vi "InsertItemByPath.vi"(8 "error in (no error)":errorcluster, 9 "ILabVIEWItem in":refnum<class "ILabVIEWItem.lvclass">, 10 "Path":string, 11 "CDependencyList in":refnum<class "CDependencyList.lvclass">) -> (0 "error out":errorcluster, 3 "CDependencyList out":refnum<class "CDependencyList.lvclass">)   [LabVIEW 2020, in "DependencyInspection.lvlib" / "CDependencyList.lvclass"]
uses:
  CDependencyList.lvclass
  obj/Addons/LabVIEWObjectInterfaces.lvlibp/LabVIEWObjectInterfaces/ILabVIEWItem/ILabVIEWItem.lvclass
  CDependencyList.lvclass/CDependencyList.ctl
  <vilib>/Utility/miscctls.llb/LVMapReplaceAction.ctl
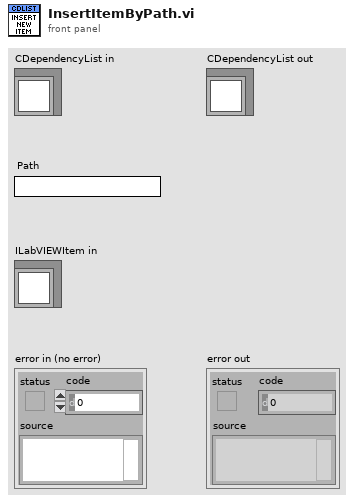
[diagram p1: front panel]
types:
  T1 = typedef "LVMapReplaceAction.ctl" = enum32{"Modify Entry only if found", "Add or Modify Entry", "Delete Entry"}
  T2 = typedef "DependencyInspection.lvlib/CDependencyList.lvclass/DependencyListRef.ctl" = refnum<data-value>
  T3 = typedef "DependencyInspection.lvlib/CDependencyList.lvclass/DependencyList.ctl" = map{string, refnum<class "ILabVIEWItem.lvclass">}
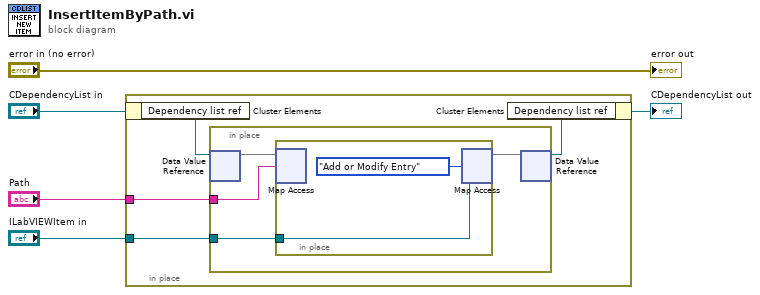
[diagram p0: block diagram]
diagram:
  n1 = in-place {
    in-place-border: "ILabVIEWItem in" -> [w9]
    in-place-border: "Path" -> [w6]
    n2 = in-place-cluster #1("CDependencyList in") -> ("Dependency list ref"=w8:T2)
    n3 = in-place {
      in-place-border: w9 -> [w13]
      in-place-border: w6 -> [w10]
      n4 = in-place-dvr #2(w8) -> (w12:T3)  [unwired: 1 out]
      n5 = in-place {
        in-place-border: w13 -> [w15]
        n6 = in-place-map #3(w12, w10) -> ()  [unwired: 1 in, 2 out]
        n7 = in-place-map #3(w15, LVMapReplaceAction."Add or Modify Entry" ("action")) -> (w11:T3)  [unwired: 2 out]
      }
      n8 = in-place-dvr #2(w11) -> (w7:T2)  [unwired: 1 out]
    }
    n9 = in-place-cluster #1("Dependency list ref"=w7) -> (→"CDependencyList out":refnum<class "CDependencyList.lvclass">)
  }
  "error out" <- "error in (no error)"
